vi "Search Cave.vi"(10 "Cave Name":string, 11 "Caves":T1[](array[typedef])) -> (1 "Index":i32, 2 "Found?":bool, 3 "Cave":T1)   [LabVIEW 2019, in "Day 12.lvlib"]
uses:
  Day 12.lvlib
  Controls/Cave.ctl
  Controls/Cave Type.ctl
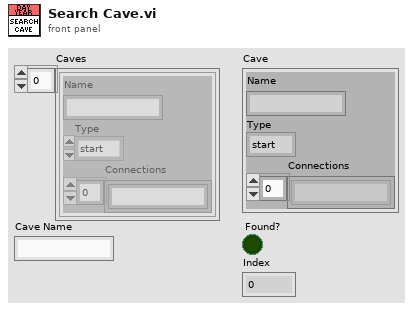
[diagram p1: front panel]
types:
  T1 = typedef "Day 12.lvlib/Cave.ctl" = cluster{"Name":string, "Type":T2, "Connections":string[]}
  T2 = typedef "Day 12.lvlib/Cave Type.ctl" = enum16{"start", "end", "small", "big"}
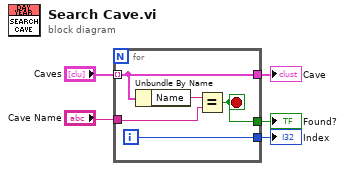
[diagram p0: block diagram]
diagram:
  n1 = for {
    tunnel: "Caves" -> [w9] mode=indexing
    tunnel: [w9] -> w3
    tunnel: "Cave Name" -> [w8]
    tunnel: [w7] -> w2
    tunnel: [w6] -> w1
    i -> [w6]
    stop <- w7 stop-if-true
    n2 = Unbundle By Name(w9) -> ("Name"=w10:string)
    n3 = Equal?(x=w10, y=w8) -> (x = y?=w7:bool)
  }
  "Cave" <- w3
  "Found?" <- w2
  "Index" <- w1
